vi "Encoder Movement.vi"(1 "Dist Error (in)":dbl) -> (0 "Speed":dbl)   [LabVIEW 2013]
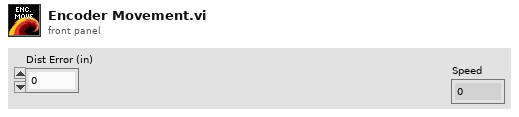
[diagram p1: front panel]
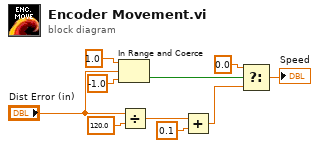
[diagram p0: block diagram]
diagram:
  n1 = In Range and Coerce(upper limit=1.0, x="Dist Error (in)", lower limit=-1.0) -> (In Range?=w3:bool)  [unwired: 1 out]
  n2 = Divide(x="Dist Error (in)", y=120.0) -> (x/y=w9:dbl)
  n3 = Add(x=w9, y=0.1) -> (x+y=w7:dbl)
  n4 = Select(t=0.0, s=w3, f=w7) -> (s? t:f=→"Speed":dbl)
